vi "RIOcardStorage.vi"(8 "Error in":errorcluster, 9 "Channel Settings":T4[][](array[typedef]), 10 "Card Settings":T1 {"Sample Rate" format="%#_3p"}, 11 "Tree DVR in":refnum<data-value>) -> (0 "error out":errorcluster)   [LabVIEW 2014]
uses:
  Controls/RIOSettingsChannelSettings.ctl
  <vilib>/MDSplus/Classes/Tree_Class/Tree.lvclass
  Controls/RIOSettingsCardSettingsArray.ctl
  Controls/RIOSettingsCardSettings.ctl
  <vilib>/userdefined/High Color/nirio_resource_hc.ctl
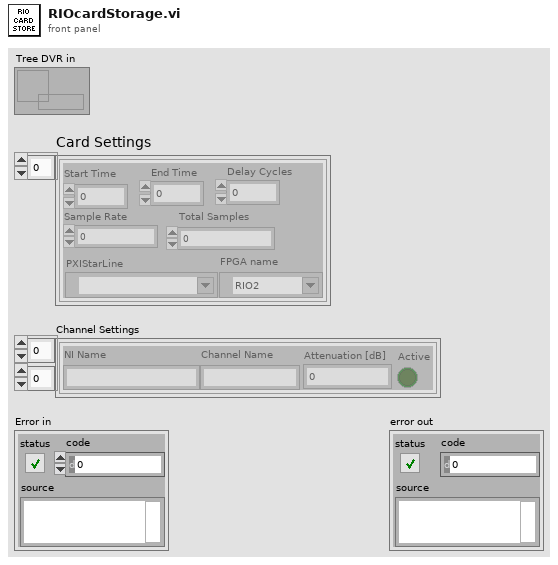
[diagram p1: front panel]
types:
  T1 = typedef "RIOSettingsCardSettingsArray.ctl" = T2[]
  T2 = typedef "RIOSettingsCardSettings.ctl" = cluster{"Start Time":dbl, "End Time":dbl, "Sample Rate":dbl, "Total Samples":u64, "PXIStarLine":tag, "Delay Cycles":u64, "FPGA name":T3}
  T3 = typedef "nirio_resource_hc.ctl" = tag
  T4 = typedef "RIOSettingsChannelSettings.ctl" = cluster{"Channel Name":string, "Active":bool, "NI Name":string, "Attenuation [dB]":i32}
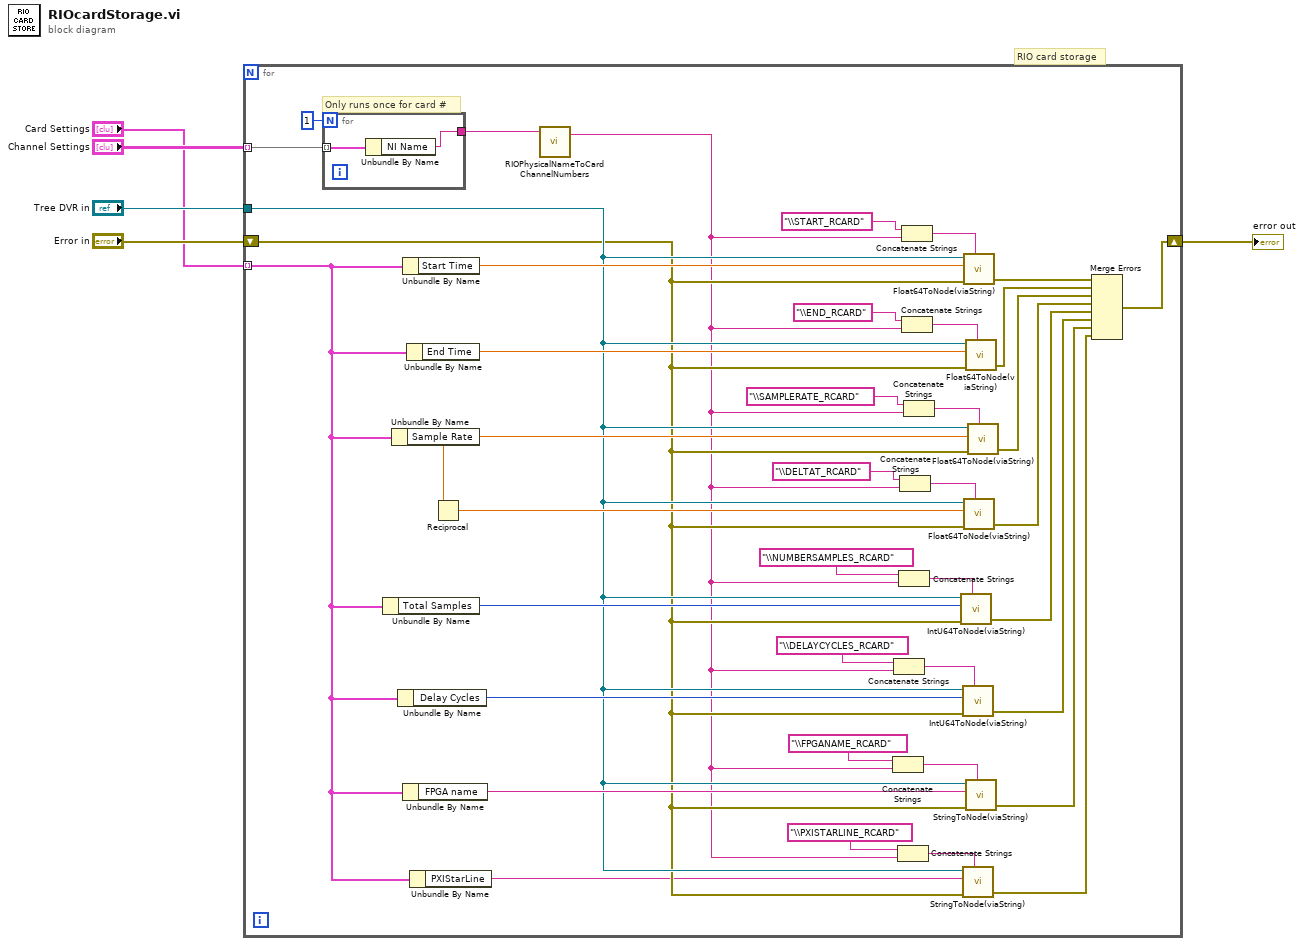
[diagram p0: block diagram]
diagram:
  # "RIO card storage"
  n1 = for {
    tunnel: "Card Settings" -> [w45] mode=indexing
    shift-right: [w39] -> w2
    shift-left: "Error in" -> [w10]
    tunnel: "Channel Settings" -> [w44] mode=indexing
    tunnel: "Tree DVR in" -> [w11]
    # "Only runs once for card #"
    n2 = for {
      N: 1 -> [_]
      tunnel: w44 -> [w47] mode=indexing
      tunnel: [w46] -> w21
      n3 = Unbundle By Name(w47) -> ("NI Name"=w46:string)
    }
    n4 = Unbundle By Name(w45) -> ("Total Samples"=w22:u64)
    n5 = Unbundle By Name(w45) -> ("Sample Rate"=w30:dbl)
    n6 = Unbundle By Name(w45) -> ("Delay Cycles"=w16:u64)
    n7 = Unbundle By Name(w45) -> ("Start Time"=w38:dbl)
    n8 = Unbundle By Name(w45) -> ("FPGA name"=w13:T3)
    n9 = Unbundle By Name(w45) -> ("End Time"=w35:dbl)
    n10 = Unbundle By Name(w45) -> ("PXIStarLine"=w9:tag)
    n11 = Reciprocal(x=w30) -> (1/x=w27:dbl)
    n12 = call "RIOPhysicalNameToCardChannelNumbers.vi"("Channel Name"=w21) -> ("Card #"=w6:string)  [unwired: 1 in, 1 out]
    n13 = Concatenate Strings("\\FPGANAME_RCARD" ("string"), w6) -> (w14:string)
    n14 = Concatenate Strings("\\DELAYCYCLES_RCARD" ("string"), w6) -> (w17:string)
    n15 = Concatenate Strings("\\PXISTARLINE_RCARD" ("string"), w6) -> (w12:string)
    n16 = Concatenate Strings("\\NUMBERSAMPLES_RCARD" ("string"), w6) -> (w25:string)
    n17 = Concatenate Strings("\\DELTAT_RCARD" ("string"), w6) -> (w28:string)
    n18 = Concatenate Strings("\\START_RCARD" ("string"), w6) -> (w41:string)
    n19 = Concatenate Strings("\\END_RCARD" ("string"), w6) -> (w36:string)
    n20 = Concatenate Strings("\\SAMPLERATE_RCARD" ("string"), w6) -> (w32:string)
    n21 = call "IntU64ToNode(viaString).vi"("Tree DVR in"=w11, "U64 in"=w22, "error in (no error)"=w10, "NodePath"=w25) -> ("error out"=w23:errorcluster)  [unwired: 3 in]
    n22 = call "IntU64ToNode(viaString).vi"("Tree DVR in"=w11, "U64 in"=w16, "error in (no error)"=w10, "NodePath"=w17) -> ("error out"=w15:errorcluster)  [unwired: 3 in]
    n23 = call "StringToNode(viaString).vi"("Tree DVR in"=w11, "String value in"=w9, "error in (no error)"=w10, "NodePath"=w12) -> ("error out"=w7:errorcluster)  [unwired: 3 in]
    n24 = call "Float64ToNode(viaString).vi"("Tree DVR in"=w11, "DBL in"=w38, "error in"=w10, "NodePath"=w41) -> ("error out"=w42:errorcluster)  [unwired: 3 in]
    n25 = call "Float64ToNode(viaString).vi"("Tree DVR in"=w11, "DBL in"=w27, "error in"=w10, "NodePath"=w28) -> ("error out"=w26:errorcluster)  [unwired: 3 in]
    n26 = call "Float64ToNode(viaString).vi"("Tree DVR in"=w11, "DBL in"=w35, "error in"=w10, "NodePath"=w36) -> ("error out"=w34:errorcluster)  [unwired: 3 in]
    n27 = call "StringToNode(viaString).vi"("Tree DVR in"=w11, "String value in"=w13, "error in (no error)"=w10, "NodePath"=w14) -> ("error out"=w8:errorcluster)  [unwired: 3 in]
    n28 = call "Float64ToNode(viaString).vi"("Tree DVR in"=w11, "DBL in"=w30, "error in"=w10, "NodePath"=w32) -> ("error out"=w31:errorcluster)  [unwired: 3 in]
    n29 = Merge Errors(w42, w34, w31, w26, w23, w15, w8, w7) -> (w39:errorcluster)
  }
  "error out" <- w2
